vi "Get All References.vi"(8 "error in (no error)":errorcluster, 11 "VI Refnum in":refnum<vi>) -> (0 "error out":errorcluster, 2 "CtlRef LUT":variant, 3 "VI Refnum out":refnum<vi>)   [LabVIEW 2013, in "SET Project Data.lvlib" / "VI Data.lvclass"]
uses:
  VI Data.lvclass
  <vilib>/Utility/traverseref.llb/TRef TravTarget.ctl
  <vilib>/Utility/traverseref.llb/VI Scripting - Traverse.lvlib
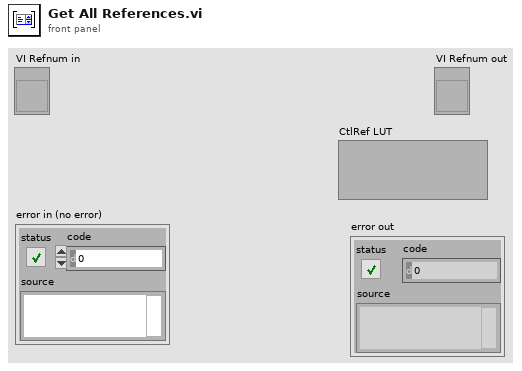
[diagram p1: front panel]
types:
  T1 = typedef "TRef TravTarget.ctl" = enum16{"FP", "BD", "Other"}
  T2 = enum32{"invalid VI type", "Standard VI", "Control VI", "Global VI", "Polymorphic VI", "Configuration VI", "SubSystem", "Facade VI", "Method VI", "Statechart Diagram VI"}
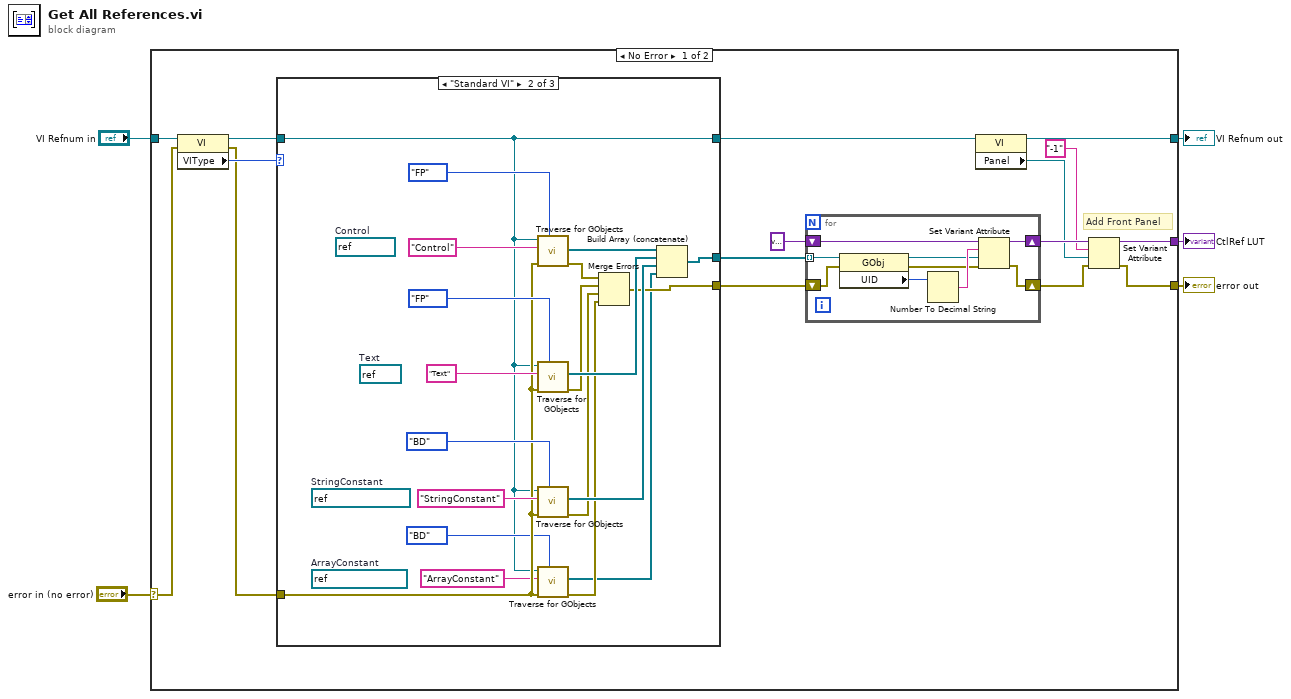
[diagram p0: block diagram]
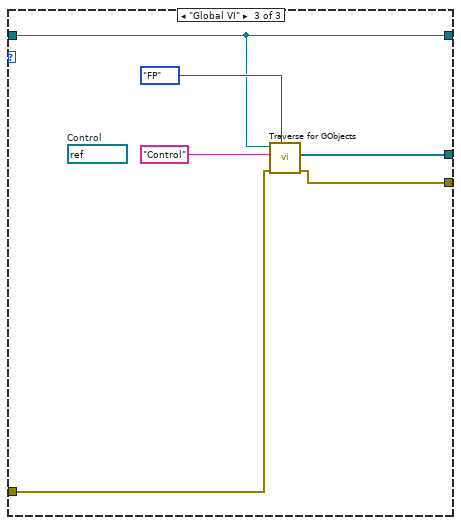
[diagram p3: hidden frame]
diagram:
  n1 = case shown="No Error" "error in (no error)" {
    selector: "error in (no error)" -> [w9 w60]
    tunnel: [w6 w60] -> w5
    tunnel: [w17 _] -> w4
    tunnel: [w16 w59] -> w3
    tunnel: "VI Refnum in" -> [w13 w59]
    frame No Error {
      # "Add Front Panel"
      n2 = property class="VI"(reference=w13, error in=w9) -> (reference out=w12:refnum<vi>, error out=w8:errorcluster, "VIType"=w11:T2)
      n3 = case shown="\"Standard VI\"" w11 {
        tunnel: [_ w43 w54] -> w21
        tunnel: [w32 w39 w53] -> w20
        tunnel: w8 -> [w32 w38 w55]
        tunnel: w12 -> [w31 w33 w56]
        tunnel: [w31 w33 w56] -> w10
        frame "invalid VI type", Default {
        }
        frame "Standard VI" {
          (unwired) refnum<vi> refnum  # ArrayConstant
          (unwired) refnum<vi> refnum  # StringConstant
          (unwired) refnum<vi> refnum  # Control
          (unwired) refnum<vi> refnum  # Text
          n4 = call <vilib>:"Traverse for GObjects.vi"("Traverse Target"=TRef_TravTarget."FP", "error in (no error)"=w38, "Class Name"="Control", "VI Refnum"=w33) -> ("error out"=w42:errorcluster, "References"=w46:refnum<vi>[])  [unwired: 4 in, 2 out]
          n5 = call <vilib>:"Traverse for GObjects.vi"("Traverse Target"=TRef_TravTarget."FP", "error in (no error)"=w38, "Class Name"="Text", "VI Refnum"=w33) -> ("error out"=w41:errorcluster, "References"=w45:refnum<vi>[])  [unwired: 4 in, 2 out]
          n6 = call <vilib>:"Traverse for GObjects.vi"("Traverse Target"=TRef_TravTarget."BD", "error in (no error)"=w38, "Class Name"="StringConstant", "VI Refnum"=w33) -> ("error out"=w40:errorcluster, "References"=w44:refnum<vi>[])  [unwired: 4 in, 2 out]
          n7 = call <vilib>:"Traverse for GObjects.vi"("Traverse Target"=TRef_TravTarget."BD", "error in (no error)"=w38, "Class Name"="ArrayConstant", "VI Refnum"=w33) -> ("error out"=w35:errorcluster, "References"=w34:refnum<vi>[])  [unwired: 4 in, 2 out]
          n8 = Merge Errors(w42, w41, w40, w35) -> (w39:errorcluster)
          n9 = Build Array (concatenate)(w46, w45, w44, w34) -> (w43:refnum<vi>[])
        }
        frame "Global VI" {
          (unwired) refnum<vi> refnum  # Control
          n10 = call <vilib>:"Traverse for GObjects.vi"("Traverse Target"=TRef_TravTarget."FP", "error in (no error)"=w55, "Class Name"="Control", "VI Refnum"=w56) -> ("error out"=w53:errorcluster, "References"=w54:refnum<vi>[])  [unwired: 4 in, 2 out]
        }
      }
      n11 = for {
        tunnel: w21 -> [w28] mode=indexing
        shift-right: [w23] -> w7
        shift-left: w20 -> [w25]
        shift-right: [w27] -> w18
        shift-left: variant ("variant") -> [w22]
        n12 = property class="GObj"(reference=w28, error in=w25) -> (reference out=w26:refnum<vi>, error out=w24:errorcluster, "UID"=w29:i32)
        n13 = Number To Decimal String(number=w29) -> (decimal integer string=w30:string)  [unwired: 1 in]
        n14 = Set Variant Attribute(Variant=w22, name=w30, value=w26, error in=w24) -> (Variant out=w27:variant, error out=w23:errorcluster)  [unwired: 1 out]
      }
      n15 = property class="VI"(reference=w10) -> (reference out=w16:refnum<vi>, "Panel"=w15:refnum<vi>)  [unwired: 1 in, 1 out]
      n16 = Set Variant Attribute(Variant=w18, name="-1", value=w15, error in=w7) -> (Variant out=w17:variant, error out=w6:errorcluster)  [unwired: 1 out]
    }
    frame Error {
    }
  }
  "CtlRef LUT" <- w4
  "VI Refnum out" <- w3
  "error out" <- w5
